vi "Longer Pump dLSP501 Fast Run.vi"() -> ()   [LabVIEW 2023, in "Longer Pump dLSP501 Series.lvlib"]
uses:
  <instrlib>/Longer Pump dLSP501 Modbus RTU Series/Longer Pump dLSP501 Series.lvlib
  <vilib>/NI/Modbus Library/API/Master/Modbus Master.lvclass
  C:/Program Files/National Instruments/LabVIEW 2023/vi.lib/NI/Modbus Library/API/Modbus API.lvclass
  <instrlib>/Longer Pump dLSP501 Modbus RTU Series/Private/Initialize - Integrated Address.vi
panel:
  out "Error out":errorcluster caption="错误输出"
  in  "Error in":errorcluster caption="错误输入"
  in  "Open Port":bool caption="打开串口"
  in  "Full Speed Config":T1={"Drive Force"=80, "Run Speed"=300, "Speed Unit"="rpm", "Full Drive Force Unit"=0} caption="全速运行参数" {"Full Drive Force Unit" items=["%"]; "Run Speed" min=100 max=300 step=1; "Drive Force" min=20 max=100 step=1}
  in  "Full Speed Control":u16(ring) caption="全速控制" items=["停止", "灌注", "抽取"]
  in  "Close Port":bool caption="关闭串口"
  in  "Send Command":bool caption="发送命令"
  in  "Comm Config.":T2={"Address"=1, "Baud Rate"=115200, "Parity"=0} caption="通讯设置" {"Parity" items=["无校验", "奇校验", "偶校验", "标记", "空格"]; "Baud Rate" items=["1200"=1200, "2400"=2400, "9600"=9600, "19200"=19200, "38400"=38400, "57600"=57600, "115200"=115200]}
  in  "VISA resource name":refnum<visa-resource-name>="COM1" caption="VISA资源名"
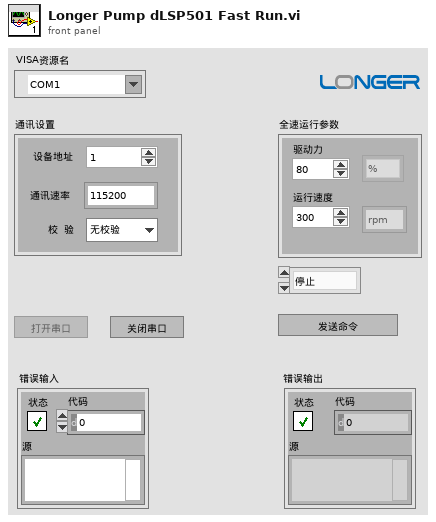
[diagram p1: front panel]
types:
  T1 = cluster{"Drive Force":u16, "Run Speed":u16, "Speed Unit":string, "Full Drive Force Unit":u16}
  T2 = cluster{"Address":u8, "Baud Rate":u32, "Parity":u16}
  T3 = enum8{"Enabled", "Disabled", "Disabled and Grayed Out"}
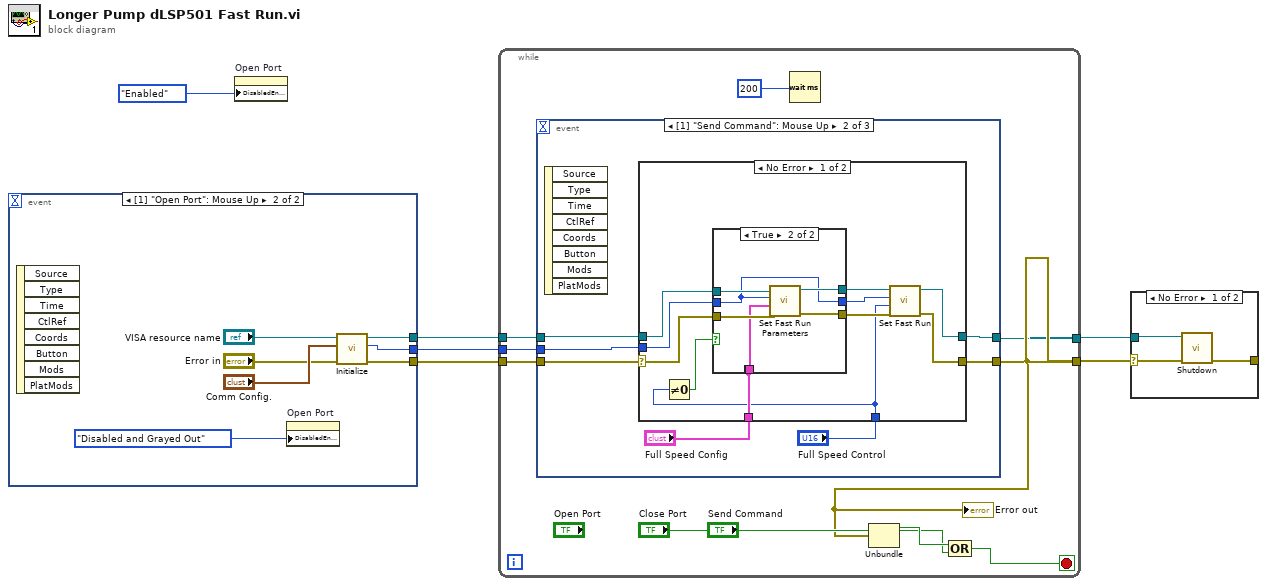
[diagram p0: block diagram]
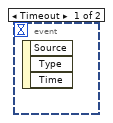
[diagram p2: hidden frame]
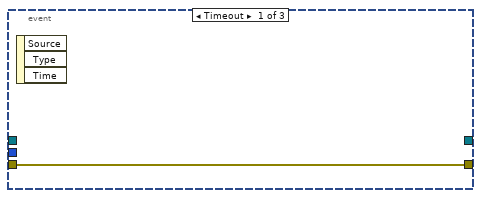
[diagram p4: hidden frame]
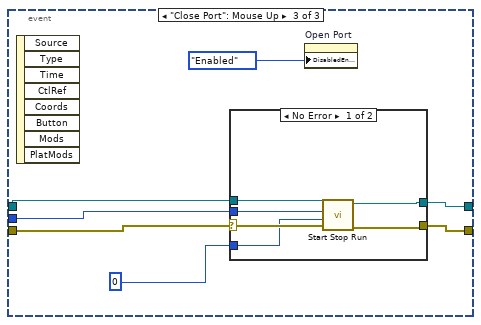
[diagram p7: hidden frame]
diagram:
  n1 = event shown="[1] \"Open Port\": Mouse Up" {
    selector: _ -> [_ _]
    dyn-events: _ -> [_ _]
    timeout: _ -> [_ _]
    tunnel: [_ w11] -> w4
    tunnel: [_ w10] -> w3
    tunnel: [_ w9] -> w2
    event Timeout {
      n2 = event-data() -> ()  [unwired: 1 in, 3 out]
    }
    event "Open Port": Mouse Up {
      n3 = event-data() -> ()  [unwired: 1 in, 8 out]
      n4 = property on="Open Port" class="Bool"("DisabledEnum"=T3."Disabled and Grayed Out" ("禁用")) -> ()  [unwired: 2 in, 2 out]
      n5 = call-poly <instrlib>:"Initialize.vi"("Error in"="Error in", "Comm. Config"="Comm Config.", "VISA resource name"="VISA resource name") -> ("Error out"=w11:errorcluster, "Channel"=w10:i32, "serial master instance"=w9:refnum<class "Modbus Master.lvclass">)  [unwired: 5 in]
    }
  }
  n6 = property on="Open Port" class="Bool"("DisabledEnum"=T3."Enabled" ("禁用")) -> ()  [unwired: 2 in, 2 out]
  n7 = while {
    tunnel: [w14] -> w6
    tunnel: [w17] -> w5
    tunnel: w4 -> [w19]
    tunnel: w2 -> [w18]
    tunnel: w3 -> [w16]
    stop <- w22 stop-if-true
    n8 = event shown="[1] \"Send Command\": Mouse Up" {
      selector: _ -> [_ _ _]
      dyn-events: _ -> [_ _ _]
      timeout: _ -> [_ _ _]
      tunnel: w19 -> [w23 w30 w59]
      tunnel: w18 -> [_ w29 w58]
      tunnel: [_ w28 w57] -> w17
      tunnel: [w23 w27 w56] -> w14
      tunnel: w16 -> [_ w26 w55]
      event Timeout {
        n9 = event-data() -> ()  [unwired: 1 in, 3 out]
      }
      event "Send Command": Mouse Up {
        n10 = event-data() -> ()  [unwired: 1 in, 8 out]
        n11 = case shown="No Error" w30 {
          selector: w30 -> [w40 w51]
          tunnel: w29 -> [w41 w52]
          tunnel: [w33 w52] -> w28
          tunnel: [w32 w51] -> w27
          tunnel: "Full Speed Control" -> [w31 _]
          tunnel: w26 -> [w39 _]
          tunnel: "Full Speed Config" -> [w37 _]
          frame No Error {
            n12 = Not Equal To 0?(x=w31) -> (x != 0?=w38:bool)
            n13 = case shown="True" w38 {
              tunnel: w41 -> [w44 w50]
              tunnel: w40 -> [w42 w49]
              tunnel: w39 -> [w43 w45]
              tunnel: w37 -> [_ _]
              tunnel: w37 -> [_ w48]
              tunnel: [w42 w46] -> w35
              tunnel: [w44 w47] -> w36
              tunnel: [w43 w45] -> w34
              frame False {
              }
              frame True {
                n14 = call <instrlib>:"Set Fast Run Parameters.vi"("Error in"=w49, "Full Speed Config"=w48, "Channel"=w45, "Modbus instance in"=w50) -> ("Error out"=w46:errorcluster, "Modbus instance out"=w47:refnum<class "Modbus Master.lvclass">)  [unwired: 6 in]
              }
            }
            n15 = call <instrlib>:"Set Fast Run.vi"("Error in"=w35, "Full Speed Control"=w31, "Channel"=w34, "Modbus instance in"=w36) -> ("Error out"=w32:errorcluster, "Modbus instance out"=w33:refnum<class "Modbus Master.lvclass">)  [unwired: 6 in]
          }
          frame Error {
          }
        }
      }
      event "Close Port": Mouse Up {
        n16 = event-data() -> ()  [unwired: 1 in, 8 out]
        n17 = case shown="No Error" w59 {
          selector: w59 -> [w64 w66]
          tunnel: w58 -> [w65 w67]
          tunnel: [w63 w67] -> w57
          tunnel: [w61 w66] -> w56
          tunnel: 0 -> [w62 _]
          tunnel: w55 -> [w60 _]
          frame No Error {
            n18 = call <instrlib>:"Start Stop Run.vi"("Error in"=w64, "Start/Stop"=w62, "Channel"=w60, "Modbus instance in"=w65) -> ("Error out"=w61:errorcluster, "Modbus instance out"=w63:refnum<class "Modbus Master.lvclass">)  [unwired: 6 in]
          }
          frame Error {
          }
        }
        n19 = property on="Open Port" class="Bool"("DisabledEnum"=T3."Enabled" ("禁用")) -> ()  [unwired: 2 in, 2 out]
      }
    }
    "Error out" <- w14
    n20 = Wait (ms)(milliseconds to wait=u32 200 ("毫秒计时值")) -> ()  [unwired: 1 out]
    n21 = Unbundle(w14) -> ("status"=w20:bool)  [unwired: 2 out]
    n22 = Compound Arithmetic op=OR ("复合运算")(w20, "Close Port") -> (w22:bool)
  }
  n23 = case shown="No Error" w6 {
    selector: w6 -> [w69 w71]
    tunnel: w5 -> [w70 _]
    tunnel: [w68 w71] -> _
    frame No Error {
      n24 = call-dynamic "Shutdown.vi"("error in"=w69, "Modbus master in"=w70) -> ("error out"=w68:errorcluster)  [unwired: 9 in]
    }
    frame Error {
    }
  }
